vi "Get All Protocols.vi"(8 "error in":errorcluster, 11 "Protocols In":refnum<class "Protocol.lvclass">[](array[class])) -> (0 "error out":errorcluster, 2 "Array":string[](array[string]), 3 "Protocols Out":refnum<class "Protocol.lvclass">[](array[class]))   [LabVIEW 2016, in "Protocol.lvclass"]
uses:
  Protocol Class/Protocol.lvclass
  Protocol Class/Protocol.lvclass/Protocol.ctl
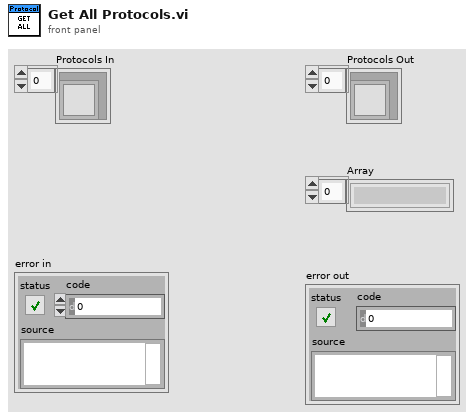
[diagram p1: front panel]
types:
  T1 = typedef "Protocol_enum_type.ctl" = enum16{"None", "MODBUS", "HART", "Fieldbus", "Profibus DP", "Profibus PA", "DeviceNET", "USB"}
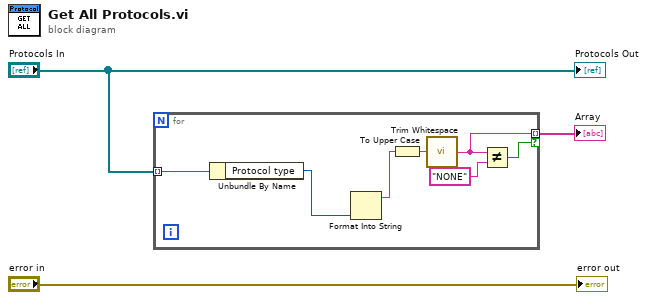
[diagram p0: block diagram]
diagram:
  n1 = for {
    tunnel: "Protocols In" -> [w10] mode=indexing
    tunnel: [w6] -> w2 mode=indexing if=w5
    n2 = Unbundle By Name(w10) -> ("Protocol type"=w4:T1)
    n3 = Format Into String(w4) -> (resulting string=w9:string)  [unwired: 3 in, 1 out]
    n4 = To Upper Case(1:w9) -> (0:w8:string)
    n5 = call <vilib>:"Trim Whitespace.vi"("string"=w8) -> ("trimmed string"=w6:string)  [unwired: 1 in]
    n6 = Not Equal?(x=w6, y="NONE") -> (x != y?=w5:bool)
  }
  "Array" <- w2
  "Protocols Out" <- "Protocols In"
  "error out" <- "error in"
